vi "WLAN - TV - RW - UTIL - CenterFrequencyToChannelNumber(wl).vi"(0 "Center Frequency(Hz)":dbl=2407000000.0, 5 "Channel BW(Hz)":dbl) -> (4 "Coherced Channel Number":i32, 6 "Coherced Center Frequency (Hz)":dbl)   [LabVIEW 2011]
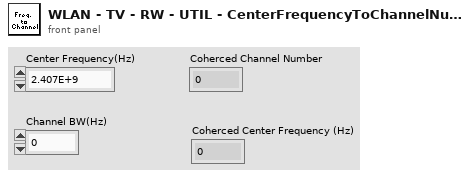
[diagram p1: front panel]
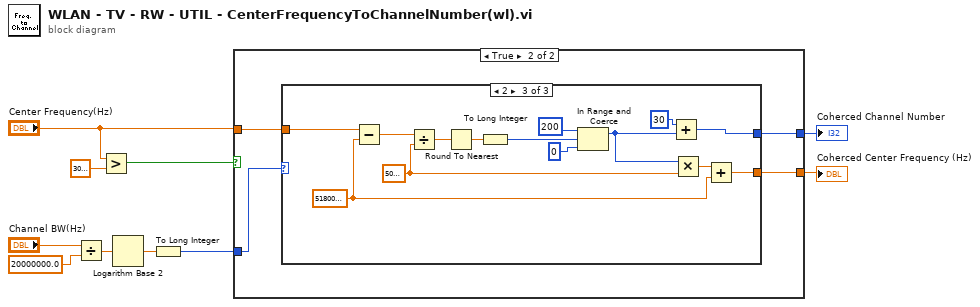
[diagram p0: block diagram]
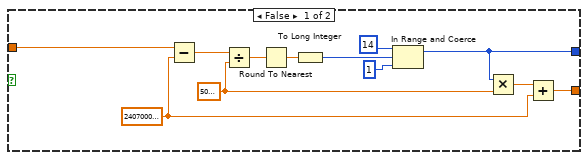
[diagram p2: hidden frame]
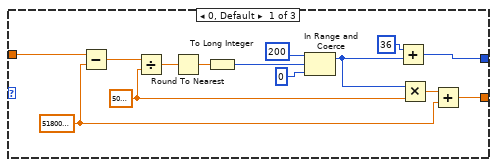
[diagram p3: hidden frame]
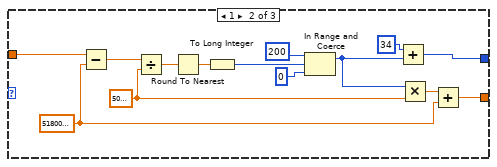
[diagram p4: hidden frame]
diagram:
  n1 = Divide(x="Channel BW(Hz)", y=20000000.0) -> (x/y=w4:dbl)
  n2 = Greater?(x="Center Frequency(Hz)", y=3000000000.0) -> (0:w2:bool)
  n3 = Logarithm Base 2(1:w4) -> (0:w3:dbl)
  n4 = To Long Integer(number=w3) -> (32bit integer=w1:i32)
  n5 = case shown="True" w2 {
    tunnel: "Center Frequency(Hz)" -> [w16 w26]
    tunnel: [w15 w24] -> w10
    tunnel: [w11 w25] -> w9
    tunnel: w1 -> [_ w23]
    frame False {
      w14 = 5000000.0 ("y")
      w12 = 2407000000.0 ("y")
      n6 = Subtract(x=w16, y=w12) -> (x-y=w22:dbl)
      n7 = Divide(x=w22, y=w14) -> (x/y=w21:dbl)
      n8 = Round To Nearest(number=w21) -> (nearest integer value=w19:dbl)
      n9 = To Long Integer(number=w19) -> (32bit integer=w20:i32)
      n10 = In Range and Coerce(upper limit=14, x=w20, lower limit=1) -> (coerced(x)=w15:i32)  [unwired: 1 out]
      n11 = Multiply(x=w15, y=w14) -> (x*y=w13:dbl)
      n12 = Add(x=w13, y=w12) -> (x+y=w11:dbl)
    }
    frame True {
      n13 = case shown="2" w23 {
        tunnel: w26 -> [w35 w49 w63]
        tunnel: [w32 w46 w60] -> w25
        tunnel: [w31 w45 w59] -> w24
        frame 0, Default {
          w34 = 5000000.0 ("y")
          w27 = 5180000000.0 ("y")
          n14 = Subtract(x=w35, y=w27) -> (x-y=w40:dbl)
          n15 = Divide(x=w40, y=w34) -> (x/y=w39:dbl)
          n16 = Round To Nearest(number=w39) -> (nearest integer value=w38:dbl)
          n17 = To Long Integer(number=w38) -> (32bit integer=w29:i32)
          n18 = In Range and Coerce(upper limit=200, x=w29, lower limit=0) -> (coerced(x)=w28:i32)  [unwired: 1 out]
          n19 = Add(x=36 ("y"), y=w28) -> (x+y=w31:i32)
          n20 = Multiply(x=w28, y=w34) -> (x*y=w33:dbl)
          n21 = Add(x=w33, y=w27) -> (x+y=w32:dbl)
        }
        frame 1 {
          w48 = 5000000.0 ("y")
          w41 = 5180000000.0 ("y")
          n22 = Subtract(x=w49, y=w41) -> (x-y=w54:dbl)
          n23 = Divide(x=w54, y=w48) -> (x/y=w53:dbl)
          n24 = Round To Nearest(number=w53) -> (nearest integer value=w52:dbl)
          n25 = To Long Integer(number=w52) -> (32bit integer=w43:i32)
          n26 = In Range and Coerce(upper limit=200, x=w43, lower limit=0) -> (coerced(x)=w42:i32)  [unwired: 1 out]
          n27 = Add(x=34 ("y"), y=w42) -> (x+y=w45:i32)
          n28 = Multiply(x=w42, y=w48) -> (x*y=w47:dbl)
          n29 = Add(x=w47, y=w41) -> (x+y=w46:dbl)
        }
        frame 2 {
          w62 = 5000000.0 ("y")
          w55 = 5180000000.0 ("y")
          n30 = Subtract(x=w63, y=w55) -> (x-y=w68:dbl)
          n31 = Divide(x=w68, y=w62) -> (x/y=w67:dbl)
          n32 = Round To Nearest(number=w67) -> (nearest integer value=w66:dbl)
          n33 = To Long Integer(number=w66) -> (32bit integer=w57:i32)
          n34 = In Range and Coerce(upper limit=200, x=w57, lower limit=0) -> (coerced(x)=w56:i32)  [unwired: 1 out]
          n35 = Add(x=30 ("y"), y=w56) -> (x+y=w59:i32)
          n36 = Multiply(x=w56, y=w62) -> (x*y=w61:dbl)
          n37 = Add(x=w61, y=w55) -> (x+y=w60:dbl)
        }
      }
    }
  }
  "Coherced Channel Number" <- w10
  "Coherced Center Frequency (Hz)" <- w9
